vi "batteryMonitor.vi"(7 "Mode":T1(ring), 8 "Error In":errorcluster, 10 "Iteration Skip":i32=100, 11 "Battery Power Reading":T2 {"Current" format="%#.3g A"; "Power" format="%#.3g W"; "Shunt Voltage" format=" %#.3g V"; "Bus Voltage" format="%#.3g V"; "Voltage (Total)" format="%#.3g V"}) -> (0 "Error Out":errorcluster, 1 "Total Capacity":dbl format="%.1f W-s", 2 "Power Used":dbl format="%.1f W-s", 3 "Battery Charge":dbl(slide) scale=0.0..100.0)   [LabVIEW 2017]
uses:
  Sensors/Power Sensor - Adafruit INA219/INA219 Measurements.ctl
  <vilib>/Utility/file.llb/Write Delimited Spreadsheet (string).vi
  <vilib>/Utility/file.llb/Read Delimited Spreadsheet (DBL).vi
panel:
  out "Write Time":u32
  out "File Location":path
  out "Written to File":string[][](array[string])
  # "Typically ~6 ms"
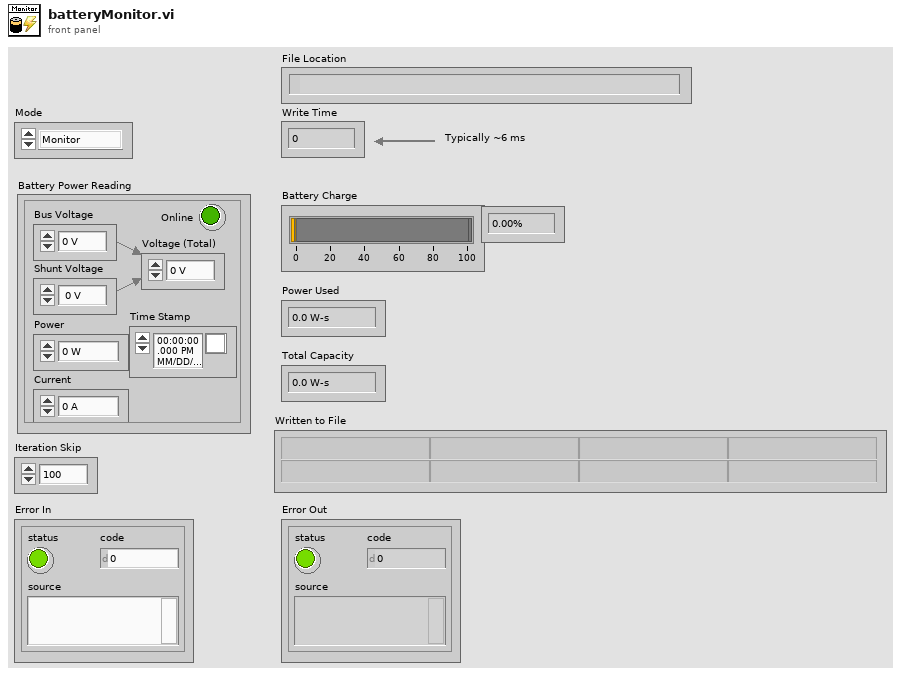
[diagram p1: front panel]
types:
  T1 = enum16{"Monitor", "Initialize", "Reset", "Write to File"}
  T2 = typedef "INA219 Measurements.ctl" = cluster{"Voltage (Total)":dbl, "Bus Voltage":dbl, "Shunt Voltage":dbl, "Power":dbl, "Current":dbl, "Online":bool, "Time Stamp":timestamp}
  T3 = cluster{"Battery Charge":dbl, "Power Used":dbl, "Total Capacity":dbl}
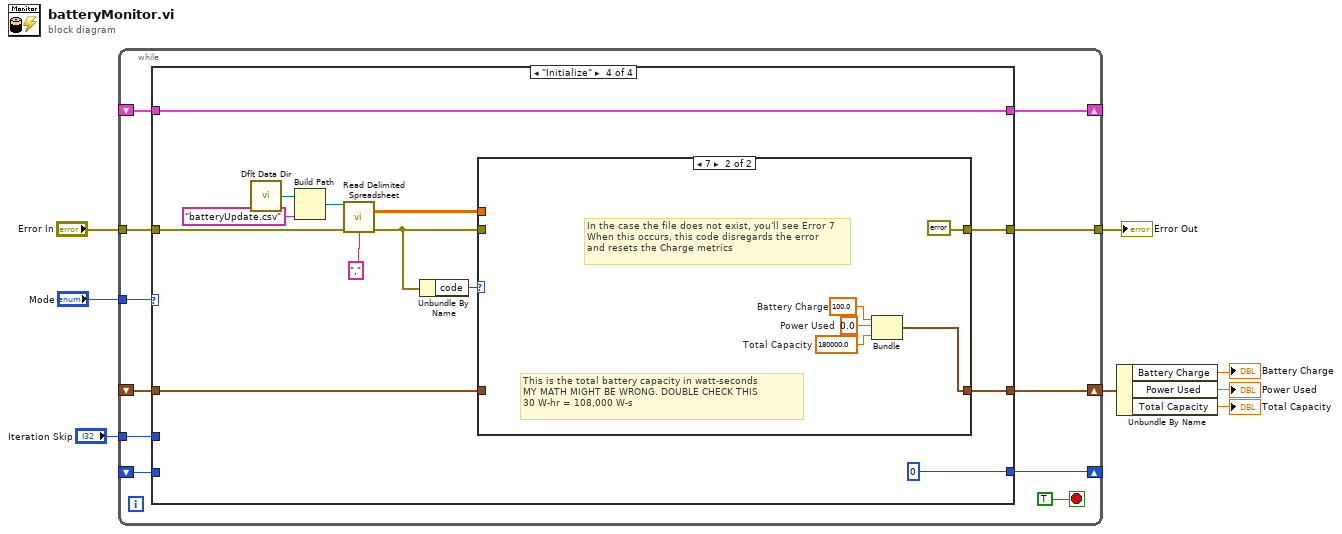
[diagram p0: block diagram]
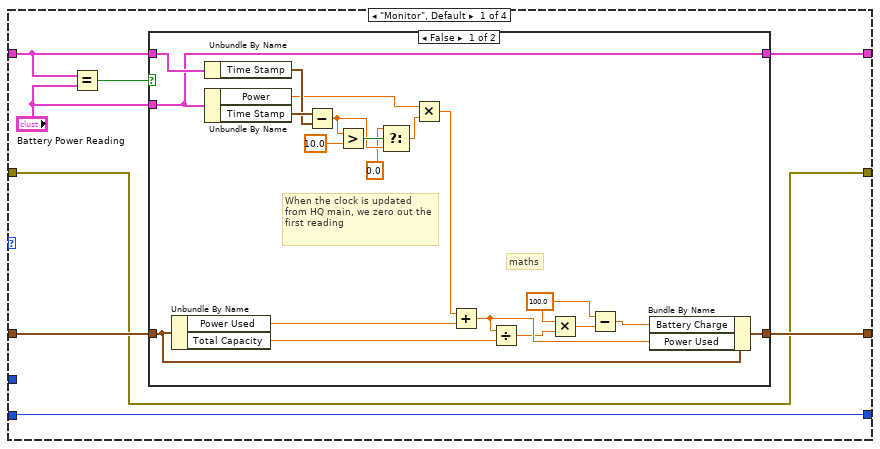
[diagram p2: hidden frame]
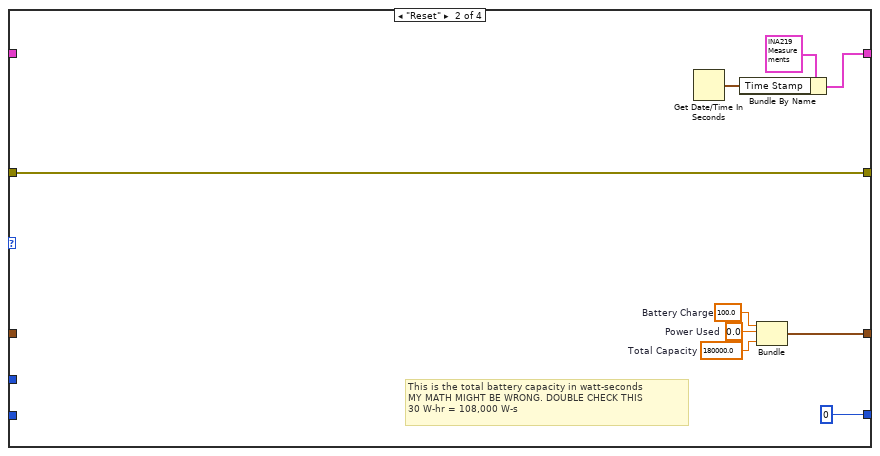
[diagram p4: hidden frame]
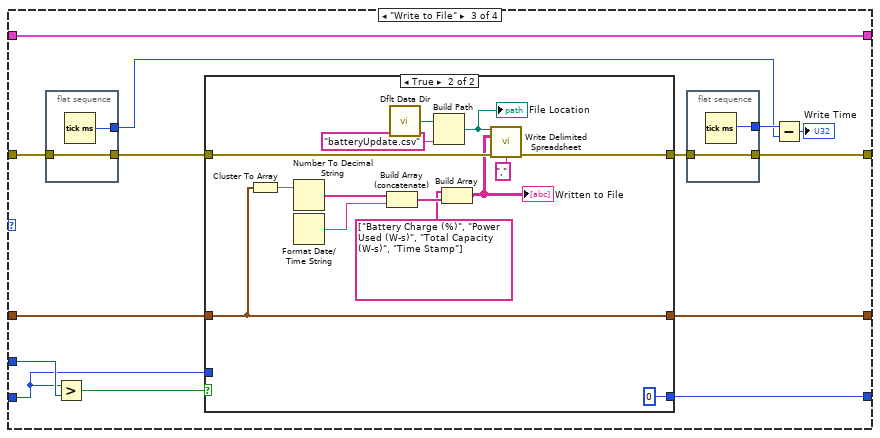
[diagram p5: hidden frame]
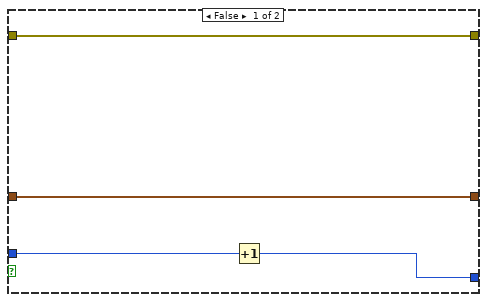
[diagram p6: hidden frame]
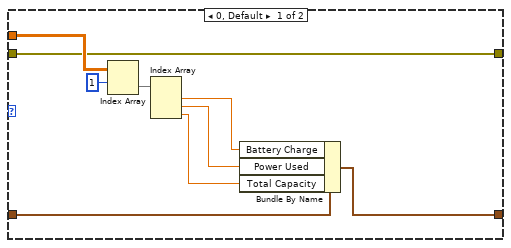
[diagram p7: hidden frame]
diagram:
  n1 = while {
    tunnel: "Mode" -> [w18]
    shift-right: [w17] -> _
    shift-left: _ -> [w16]
    shift-right: [w15] -> w7
    shift-left: _ -> [w14]
    tunnel: "Iteration Skip" -> [w13]
    shift-right: [w12] -> _
    shift-left: _ -> [w11]
    tunnel: [w10] -> w2
    tunnel: "Error In" -> [w9]
    stop <- TRUE stop-if-true
    n2 = case shown="\"Initialize\"" w18 {
      tunnel: [w27 w52 w72 w107] -> w17
      tunnel: w16 -> [w26 _ w72 w107]
      tunnel: [w22 w55 w68 w98] -> w15
      tunnel: w14 -> [w23 _ w69 w100]
      tunnel: w13 -> [_ _ w71 _]
      tunnel: [w21 0 ("Iteration Skip") w67 0 ("Iteration Skip")] -> w12
      tunnel: w11 -> [w21 _ w66 _]
      tunnel: [w20 w50 w62 w95] -> w10
      tunnel: w9 -> [w20 w50 w65 w99]
      frame "Monitor", Default {
        n3 = Equal?(x=w26, y="Battery Power Reading") -> (x = y?=w24:bool)
        n4 = case shown="False" w24 {
          tunnel: "Battery Power Reading" -> [w46 _]
          tunnel: [w46 w49] -> w27
          tunnel: w26 -> [w47 w49]
          tunnel: w23 -> [w42 w48]
          tunnel: [w41 w48] -> w22
          frame False {
            w34 = 100.0 ("x")
            # "When the clock is updated from HQ main, we zero out the first reading"
            # "maths"
            n5 = Unbundle By Name(w42) -> ("Power Used"=w40:dbl, "Total Capacity"=w37:dbl)
            n6 = Unbundle By Name(w47) -> ("Time Stamp"=w44:timestamp)
            n7 = Unbundle By Name(w46) -> ("Power"=w43:dbl, "Time Stamp"=w45:timestamp)
            n8 = Subtract(x=w45, y=w44) -> (x-y=w30:dbl)
            n9 = Greater?(x=w30, y=10.0) -> (0:w31:bool)
            n10 = Select(t=0.0 ("y"), s=w31, f=w30) -> (s? t:f=w28:dbl)
            n11 = Multiply(x=w43, y=w28) -> (x*y=w39:dbl)
            n12 = Add(x=w39, y=w40) -> (x+y=w38:dbl)
            n13 = Divide(x=w38, y=w37) -> (x/y=w36:dbl)
            n14 = Multiply(x=w34, y=w36) -> (x*y=w35:dbl)
            n15 = Subtract(x=w34, y=w35) -> (x-y=w33:dbl)
            n16 = Bundle By Name(cluster=w42, "Battery Charge"=w33, "Power Used"=w38) -> (w41:T3)
          }
          frame True {
            # "When the latest battery reading is identical to the last (which happens when this VI runs more often than the power readings), skip processing and pass along values"
          }
        }
      }
      frame "Reset" {
        w56 = 180000.0  # Total Capacity
        w57 = 0.0  # Power Used
        w58 = 100.0  # Battery Charge
        # "This is the total battery capacity in watt-seconds\nMY MATH MIGHT BE WRONG. DOUBLE CHECK THIS\n30 W-hr = 108,000 W-s"
        n17 = Get Date/Time In Seconds() -> (seconds since 1Jan1904=w53:timestamp)
        n18 = Bundle By Name(cluster=T2 {"Voltage (Total)"=0.0, "Bus Voltage"=0.0, "Shunt Voltage"=0.0, "Power"=0.0, "Current"=0.0, "Online"=FALSE, "Time Stamp"=timestamp(0 s since 1904-01-01)} ("Battery Power Reading"), "Time Stamp"=w53) -> (w52:T2)
        n19 = Bundle("Battery Charge"=w58, "Power Used"=w57, "Total Capacity"=w56) -> (w55:T3)  [unwired: 1 in]
      }
      frame "Write to File" {
        n20 = flat-sequence {
          tunnel: w65 -> [w76]
          tunnel: [w76] -> w64
          tunnel: [w75] -> w60
          frame #0 {
            n21 = Tick Count (ms)() -> (millisecond timer value=w75:u32)
          }
        }
        n22 = Greater?(x=w66, y=w71) -> (0:w70:bool)
        n23 = case shown="True" w70 {
          tunnel: w69 -> [w80 w91]
          tunnel: [w80 w91] -> w68
          tunnel: [w78 0] -> w67
          tunnel: w66 -> [w79 _]
          tunnel: [w77 w84] -> w63
          tunnel: w64 -> [w77 w83]
          frame False {
            n24 = Increment(x=w79) -> (x+1=w78:i32)
          }
          frame True {
            n25 = Cluster To Array(cluster=w91) -> (array=w94:dbl[])
            n26 = Number To Decimal String(number=w94) -> (decimal integer string=w93:string[])  [unwired: 1 in]
            n27 = Format Date/Time String() -> (date/time string=w92:string)  [unwired: 3 in]
            n28 = Build Array (concatenate)(w93, w92) -> (w89:string[])
            n29 = call <vilib>:"Dflt Data Dir.vi"() -> ("App:Default Data Directory"=w86:path)
            n30 = Build Path(base path=w86, name or relative path="batteryUpdate.csv") -> (appended path=w87:path)
            "File Location" <- w87
            n31 = Build Array(string[] ["Battery Charge (%)", "Power Used (W-s)", "Total Capacity (W-s)", "Time Stamp"], w89) -> (w81:string[][])
            "Written to File" <- w81
            n32 = call-poly <vilib>:"Write Delimited Spreadsheet.vi"("file path (dialog if empty)"=w87, "2D data"=w81, "error in (no error)"=w83, "delimiter (\\t)"="," ("delimiter (\\t)")) -> ("error out"=w84:errorcluster)  [unwired: 10 in, 1 out]
          }
        }
        n33 = flat-sequence {
          tunnel: w63 -> [w74]
          tunnel: [w74] -> w62
          tunnel: [w73] -> w61
          frame #0 {
            n34 = Tick Count (ms)() -> (millisecond timer value=w73:u32)
          }
        }
        n35 = Subtract(x=w61, y=w60) -> (x-y=→"Write Time":u32)
      }
      frame "Initialize" {
        n36 = call <vilib>:"Dflt Data Dir.vi"() -> ("App:Default Data Directory"=w105:path)
        n37 = Build Path(base path=w105, name or relative path="batteryUpdate.csv") -> (appended path=w102:path)
        n38 = call-poly <vilib>:"Read Delimited Spreadsheet.vi"("file path (dialog if empty)"=w102, "error in (no error)"=w99, "delimiter (\\t)"="," ("delimiter (\\t)")) -> ("all rows"=w101:dbl[][], "error out"=w96:errorcluster)  [unwired: 7 in, 4 out]
        n39 = Unbundle By Name(w96) -> ("code"=w97:i32)
        n40 = case shown="7" w97 {
          tunnel: w101 -> [w116 _]
          tunnel: w100 -> [w114 _]
          tunnel: [w109 w117] -> w98
          tunnel: w96 -> [w108 _]
          tunnel: [w108 errorcluster {"status"=FALSE, "code"=0, "source"=""} ("error out")] -> w95
          frame 0, Default {
            n41 = Index Array(array=w116, index (row)=1) -> (element=w113:dbl[])  [unwired: 1 in]
            n42 = Index Array(array=w113) -> (element #1=w110:dbl, element #2=w111:dbl, element #3=w112:dbl)  [unwired: 3 in]
            n43 = Bundle By Name(cluster=w114, "Battery Charge"=w110, "Power Used"=w111, "Total Capacity"=w112) -> (w109:T3)
          }
          frame 7 {
            w118 = 180000.0  # Total Capacity
            w119 = 0.0  # Power Used
            w120 = 100.0  # Battery Charge
            # "In the case the file does not exist, you'll see Error 7\nWhen this occurs, this code disregards the error\nand resets the Charge metrics"
            # "This is the total battery capacity in watt-seconds\nMY MATH MIGHT BE WRONG. DOUBLE CHECK THIS\n30 W-hr = 108,000 W-s"
            n44 = Bundle("Battery Charge"=w120, "Power Used"=w119, "Total Capacity"=w118) -> (w117:T3)  [unwired: 1 in]
          }
        }
      }
    }
  }
  "Error Out" <- w2
  n45 = Unbundle By Name(w7) -> ("Battery Charge"=→"Battery Charge":dbl, "Power Used"=→"Power Used":dbl, "Total Capacity"=→"Total Capacity":dbl)
